vi "Change10000.vi"(8 "error in":errorcluster, 11 "Input":T1(array[cluster])) -> (0 "error out":errorcluster, 3 "Output data array":T1(array[cluster]))   [LabVIEW 2014]
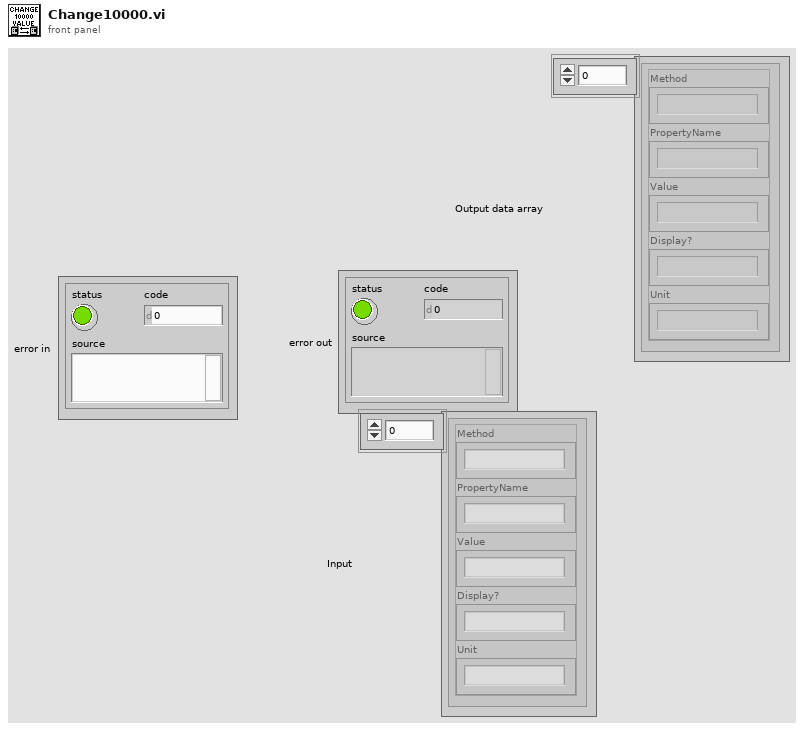
[diagram p1: front panel]
types:
  T1 = cluster{"Method":string, "PropertyName":string, "Value":string, "Display?":string, "Unit":string}[]
  T2 = cluster{"Method":string, "PropertyName":string, "Value":string, "Display?":string, "Unit":string}
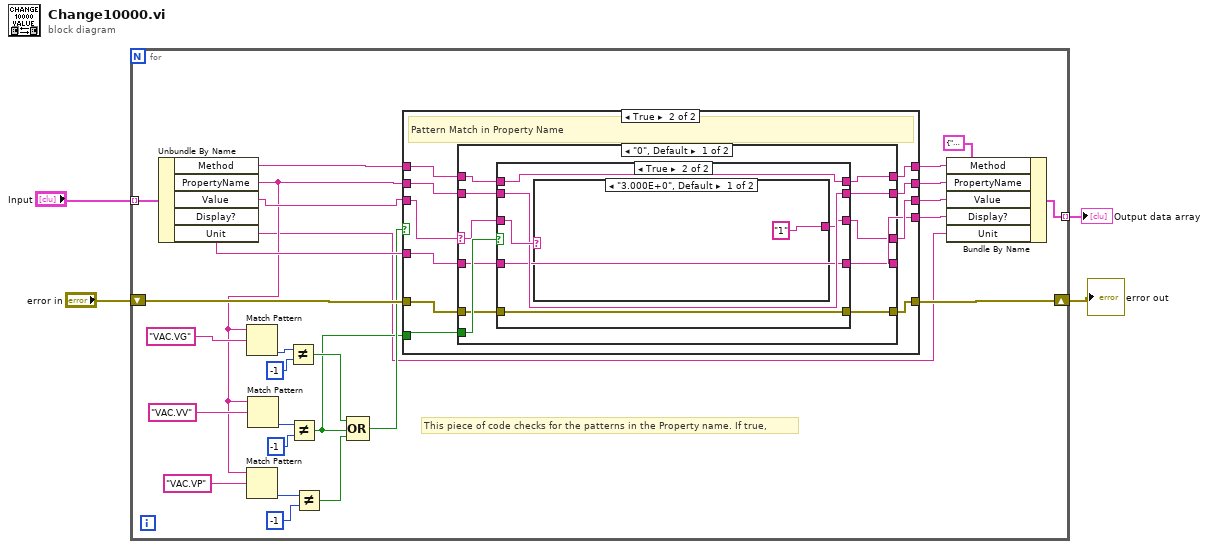
[diagram p0: block diagram]
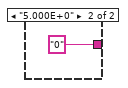
[diagram p4: hidden frame]
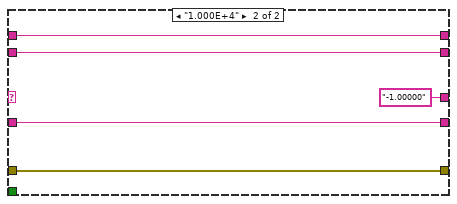
[diagram p5: hidden frame]
diagram:
  n1 = for {
    tunnel: "Input" -> [w31] mode=indexing
    shift-right: [w22] -> w3
    shift-left: "error in" -> [w12]
    tunnel: [w5] -> w1 mode=indexing
    # "This piece of code checks for the patterns in the Property name. If true,"
    n2 = Unbundle By Name(w31) -> ("Method"=w27:string, "PropertyName"=w11:string, "Value"=w30:string, "Display?"=w25:string, "Unit"=w6:string)
    n3 = Match Pattern(string=w11, regular expression="VAC.VG") -> (offset past match=w20:i32)  [unwired: 1 in, 3 out]
    n4 = Match Pattern(string=w11, regular expression="VAC.VP") -> (offset past match=w15:i32)  [unwired: 1 in, 3 out]
    n5 = Match Pattern(string=w11, regular expression="VAC.VV") -> (offset past match=w17:i32)  [unwired: 1 in, 3 out]
    n6 = Not Equal?(x=w20, y=-1) -> (x != y?=w9:bool)
    n7 = Not Equal?(x=w17, y=-1) -> (x != y?=w7:bool)
    n8 = Not Equal?(x=w15, y=-1) -> (x != y?=w10:bool)
    n9 = Compound Arithmetic op=OR(w9, w7, w10) -> (w8:bool)
    n10 = case shown="True" w8 {
      tunnel: w30 -> [w34 w47]
      tunnel: [w34 w46] -> w28
      tunnel: w27 -> [w36 w45]
      tunnel: [w36 w44] -> w26
      tunnel: w11 -> [w35 w43]
      tunnel: w25 -> [w33 w42]
      tunnel: [w33 w41] -> w24
      tunnel: [w35 w40] -> w23
      tunnel: w12 -> [w32 w39]
      tunnel: [w32 w38] -> w22
      tunnel: w7 -> [_ w37]
      frame False {
        # "Not a VAC.VG, VAC.VV, VAC.VP element"
      }
      frame True {
        # "Pattern Match in Property Name"
        n11 = case shown="\"0\", Default" w47 {
          selector: w47 -> [w55 _]
          tunnel: [w50 "-1.00000"] -> w46
          tunnel: w45 -> [w54 w75]
          tunnel: [w53 w75] -> w44
          tunnel: w43 -> [w52 w74]
          tunnel: w42 -> [w49 w73]
          tunnel: [w48 w73] -> w41
          tunnel: [w51 w74] -> w40
          tunnel: w39 -> [w57 w72]
          tunnel: [w56 w72] -> w38
          tunnel: w37 -> [w58 _]
          frame "0", Default {
            n12 = case shown="True" w58 {
              tunnel: w57 -> [w63 w69]
              tunnel: [w63 w69] -> w56
              tunnel: w55 -> [w60 w68]
              tunnel: w54 -> [w62 w67]
              tunnel: [w62 w67] -> w53
              tunnel: w52 -> [w61 w66]
              tunnel: [w61 w66] -> w51
              tunnel: [w60 w65] -> w50
              tunnel: w49 -> [w59 w64]
              tunnel: [w59 w64] -> w48
              frame False {
              }
              frame True {
                n13 = case shown="\"3.000E+0\", Default" w68 {
                  tunnel: ["1" "0"] -> w65
                  frame "3.000E+0", Default {
                  }
                  frame "5.000E+0" {
                  }
                }
              }
            }
          }
          frame "1.000E+4" {
          }
        }
      }
    }
    n14 = Bundle By Name(cluster=T2 {"Method"="", "PropertyName"="", "Value"="", "Display?"="", "Unit"=""} ("input cluster"), "Method"=w26, "PropertyName"=w23, "Value"=w28, "Display?"=w24, "Unit"=w6) -> (w5:T2)
  }
  "error out" <- w3
  "Output data array" <- w1
